vi "3dgraph.vi"() -> ()   [LabVIEW 2020]
uses:
  <vilib>/Native 3D Graph/xcontrol/3DPC_SurfacePlot.xctl
panel:
  out "3D Graph":refnum<class "Base Datatype.lvclass">[](xcontrol)
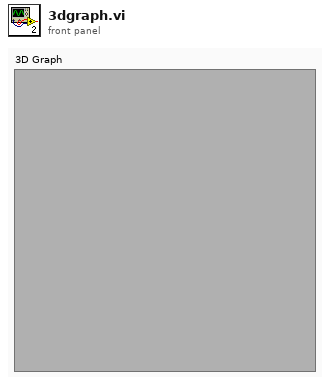
[diagram p1: front panel]
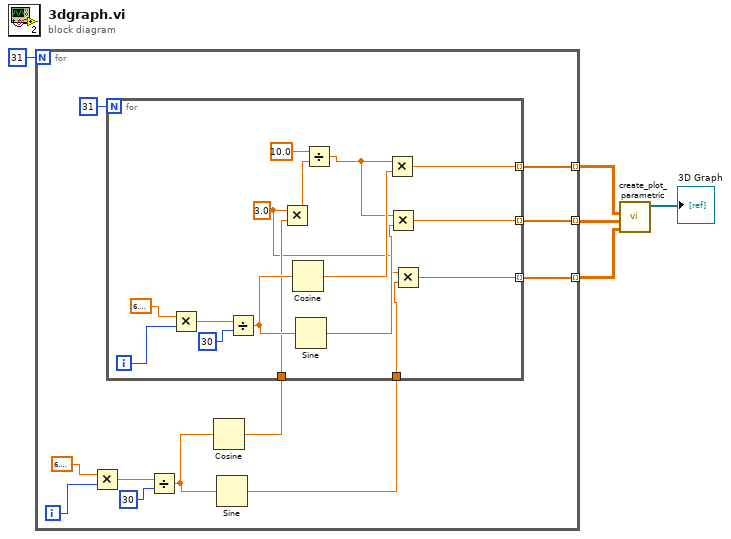
[diagram p0: block diagram]
diagram:
  n1 = for {
    N: 31 -> [_]
    tunnel: [w8] -> w2 mode=indexing
    tunnel: [w7] -> w3 mode=indexing
    tunnel: [w6] -> w1 mode=indexing
    i -> [w15]
    n2 = Multiply(x=6.283185307179586, y=w15) -> (x*y=w13:dbl)
    n3 = Divide(x=w13, y=30) -> (x/y=w11:dbl)
    n4 = Cosine(x=w11) -> (cos(x)=w10:dbl)
    n5 = Sine(x=w11) -> (sin(x)=w9:dbl)
    n6 = for {
      N: 31 -> [_]
      tunnel: w10 -> [w25]
      tunnel: w9 -> [w20]
      tunnel: [w19] -> w7 mode=indexing
      tunnel: [w18] -> w8 mode=indexing
      tunnel: [w17] -> w6 mode=indexing
      i -> [w28]
      w21 = 3.0 ("x")
      n7 = Multiply(x=6.283185307179586, y=w28) -> (x*y=w30:dbl)
      n8 = Divide(x=w30, y=30) -> (x/y=w32:dbl)
      n9 = Multiply(x=w21, y=w25) -> (x*y=w26:dbl)
      n10 = Cosine(x=w32) -> (cos(x)=w24:dbl)
      n11 = Sine(x=w32) -> (sin(x)=w22:dbl)
      n12 = Divide(x=10.0, y=w26) -> (x/y=w23:dbl)
      n13 = Multiply(x=w23, y=w24) -> (x*y=w19:dbl)
      n14 = Multiply(x=w23, y=w22) -> (x*y=w18:dbl)
      n15 = Multiply(x=w21, y=w20) -> (x*y=w17:dbl)
    }
  }
  n16 = call <vilib>:"create_plot_parametric.vi"("z matrix"=w1, "y matrix"=w2, "x matrix"=w3) -> ("plots out"=→"3D Graph":refnum<class "Base Datatype.lvclass">[])  [unwired: 2 in, 6 out]
